vi "SaveArraytoColorImageAVI.vi"() -> ()   [LabVIEW 2017]
doc: "The Sequence and Save to AVI VI acquires multiple images, displays the images in an array of image controls, and saves the sequence of images to an AVI file. A sequence is appropriate for applications that perform processing on multiple images. You can configure a sequence to acquire every frame or to skip a variable number of frames between each image. Use an AVI file to save multiple images to a single file for post-processing or to record images. \n\nIMAQ Create creates multiple image buffers. The array of image buffers is wired to IMAQ Sequence. The Skip Table input to IMAQ Sequence specifies the number of frames to skip between captures. IMAQ Sequence acquires and returns the images. An image control displays the array of images on the front panel. IMAQ Sequence performs a synchronous acquisition. To acquire asynchronously, refer to the LL Sequence VI in the IMAQ Low Level.llb.\n\nIMAQ AVI Create initializes the AVI file, IMAQ AVI Write Frame adds each image to the AVI file, and IMAQ AVI Close completes writing to the AVI file. Call IMAQ AVI Create for each AVI file created."
uses:
  <vilib>/vision/driver/NI_Vision_Acquisition_Software.lvlib
panel:
  in  "Frames Per Second":u32=30
  out "Selected Path":path
  out "Image Array":T1[](array[plugin-control])
  in  "stop":bool
  in  "Interface Name":string="cam0"
  in  "Number of images":i32=10
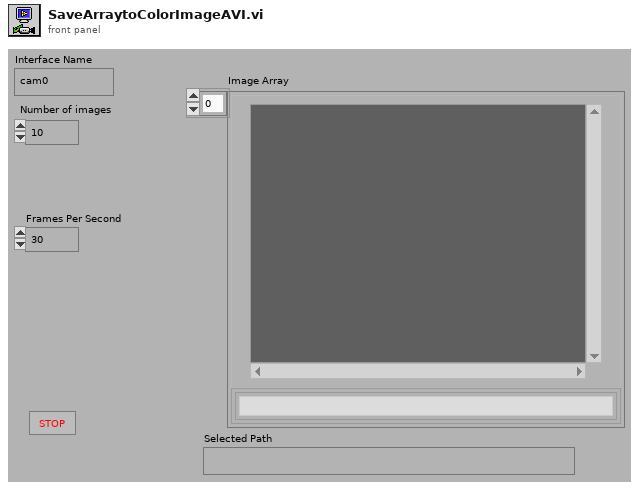
[diagram p1: front panel]
types:
  T1 = typedef "IMAQ Image.ctl" = refnum<image>
  T2 = typedef "Image Type" = u32
  T3 = enum32{"existing file", "new file", "new or existing file", "existing dir", "new dir", "new or existing dir", "existing file (use LLBs)", "new file (use LLBs)", "new or existing file (use LLBs)", "new or existing file or directory (use LLBs)"}
  T4 = typedef "IMAQdx.ctl" = refnum<k21>
  T5 = typedef "AviRefnum.ctl" = refnum<k1>
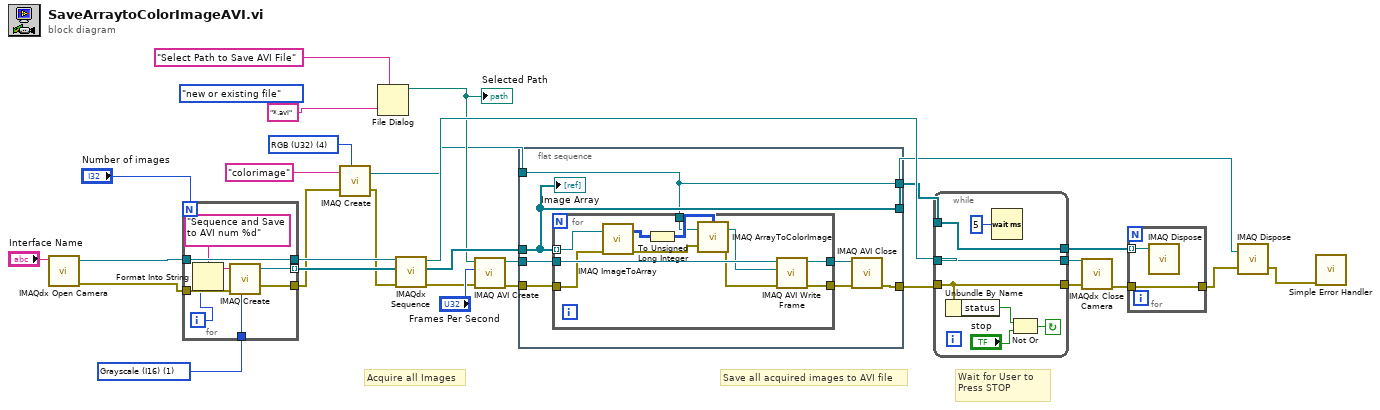
[diagram p0: block diagram]
diagram:
  w3 = T2 4 items=["Grayscale (U8)", "Grayscale (I16)", "Grayscale (SGL)", "Complex (CSG)", "RGB (U32)", "HSL (U32)", "RGB (U64)"] ("Image Type")
  w9 = T2 1 items=["Grayscale (U8)", "Grayscale (I16)", "Grayscale (SGL)", "Complex (CSG)", "RGB (U32)", "HSL (U32)", "RGB (U64)"] ("Image Type")
  (unwired) T3."new or existing file" ("select mode (2)")
  # "Acquire all Images"
  # "Save all acquired images to AVI file"
  # "Wait for User to Press STOP"
  n1 = call <vilib>:"IMAQdx Open Camera.vi"("Session In"="Interface Name") -> ("error out"=w12:errorcluster, "Session Out"=w11:T4)  [unwired: 9 in]
  n2 = for {
    N: "Number of images" -> [_]
    tunnel: [w38] -> w2
    tunnel: [w37] -> w30 mode=indexing
    tunnel: w12 -> [w36]
    tunnel: w11 -> [w35]
    tunnel: [w35] -> w10
    tunnel: w9 -> [w31]
    i -> [w33]
    n3 = Format Into String(format string="Sequence and Save to AVI num %d", w33) -> (resulting string=w34:string)  [unwired: 2 in, 1 out]
    n4 = call "IMAQ Create"("Image Name"=w34, "Image Type"=w31, "error in (no error)"=w36) -> ("New Image"=w37:T1, "error out"=w38:errorcluster)  [unwired: 2 in]
  }
  n5 = call "IMAQ Create"("Image Name"="colorimage", "Image Type"=w3, "error in (no error)"=w2) -> ("New Image"=w7:T1, "error out"=w1:errorcluster)  [unwired: 2 in]
  n6 = File Dialog(6:"*.avi" ("pattern"), 7:"Select Path to Save AVI File" ("prompt")) -> (3:w14:path)  [unwired: 5 in, 3 out]
  "Selected Path" <- w14
  n7 = call <vilib>:"IMAQdx Sequence.vi"("error in"=w1, "Images In"=w30, "Session In"=w10) -> ("error out"=w21:errorcluster, "Images Out"=w17:T1[], "Session Out"=w16:T4)  [unwired: 6 in]
  n8 = call "IMAQ AVI Create"("error in (no error)"=w21, "Frames Per Second"="Frames Per Second", "AVI Path"=w14) -> ("error out"=w20:errorcluster, "Avi Refnum"=w22:T5)  [unwired: 7 in]
  n9 = flat-sequence {
    tunnel: [w41] -> w15
    tunnel: w22 -> [w45]
    tunnel: w20 -> [w44]
    tunnel: w17 -> [w41]
    tunnel: [w40] -> w13
    tunnel: w7 -> [w39]
    tunnel: [w39] -> w4
    frame #0 {
      n10 = for {
        tunnel: w45 -> [w56]
        tunnel: w44 -> [w48]
        tunnel: [w55] -> w42
        tunnel: [w54] -> w43
        tunnel: w41 -> [w53] mode=indexing
        tunnel: w39 -> [w50]
        n11 = call "IMAQ ImageToArray"("error in (no error)"=w48, "Image"=w53) -> ("error out"=w47:errorcluster, "Image Pixels (I16)"=w52:i16[][])  [unwired: 2 in, 3 out]
        n12 = To Unsigned Long Integer(number=w52) -> (unsigned 32bit integer=w51:u32[][])
        n13 = call "IMAQ ArrayToColorImage"("Image Pixels (U32)"=w51, "Image"=w50, "error in (no error)"=w47) -> ("Image Out"=w49:T1, "error out"=w46:errorcluster)  [unwired: 2 in]
        n14 = call "IMAQ AVI Write Frame"("error in (no error)"=w46, "Image"=w49, "Avi Refnum"=w56) -> ("error out"=w54:errorcluster, "Avi Refnum (duplicate)"=w55:T5)  [unwired: 7 in]
      }
      n15 = call "IMAQ AVI Close"("error in (no error)"=w43, "Avi Refnum"=w42) -> ("error out"=w40:errorcluster)  [unwired: 9 in]
      "Image Array" <- w41
    }
  }
  n16 = while {
    tunnel: w16 -> [w63]
    tunnel: w13 -> [w60]
    tunnel: [w60] -> w26
    tunnel: [w63] -> w25
    tunnel: [w61] -> w24
    tunnel: w15 -> [w61]
    stop <- w57 continue-if-true
    n17 = Unbundle By Name(w60) -> ("status"=w58:bool)
    n18 = Wait (ms)(milliseconds to wait=u32 5) -> ()  [unwired: 1 out]
    n19 = Not Or(1:"stop", 2:w58) -> (0:w57:bool)
  }
  n20 = call <vilib>:"IMAQdx Close Camera.vi"("error in"=w26, "Session In"=w25) -> ("error out"=w28:errorcluster)  [unwired: 9 in]
  n21 = for {
    tunnel: w28 -> [w65]
    tunnel: [w65] -> w6
    tunnel: w24 -> [w64] mode=indexing
    n22 = call "IMAQ Dispose"("Image"=w64) -> ()  [unwired: 5 in, 1 out]
  }
  n23 = call "IMAQ Dispose"("Image"=w4, "error in (no error)"=w6) -> ("error out"=w5:errorcluster)  [unwired: 4 in]
  n24 = call <vilib>:"Simple Error Handler.vi"("error in (no error)"=w5) -> ()  [unwired: 4 in, 5 out]
